vi "HDF5_Test9-openFile.vi"() -> ()   [LabVIEW 2018]
uses:
  <vilib>/addons/h5labview2/base/h5o_type.ctl
  HDF5/HDF5_NoiseInfoClust.ctl
  <vilib>/addons/h5labview2/file/H5Fmode.ctl
  HDF5/lib_path_mod_20200519.vi
  <vilib>/addons/h5labview2/base/H5Equery.vi
  <vilib>/addons/h5labview2/dataset/H5Dread.llb/H5Dread.xnode
  <vilib>/addons/h5labview2/file/H5F.lvlib
  <vilib>/addons/h5labview2/group/H5G.lvlib
  <vilib>/addons/h5labview2/base/hid_t_renamed.ctl
panel:
  out "data 2":T1[][](array[typedef]) {"Sum" format="%^#.1g"}
  out "types 2":T2[](array[typedef])
  out "element":string
  out "data":T1={"Timestring"="", "Timestamp"=0.0, "df"=7629.39453125, "Sum"=0.0} {"Sum" format="%^#.1g"}
  out "found?":bool
  out "names 2":string[](array[string])
  in  "index":i32
  in  "path":path
  out "types":T2[](array[typedef])
  out "names":string[](array[string])
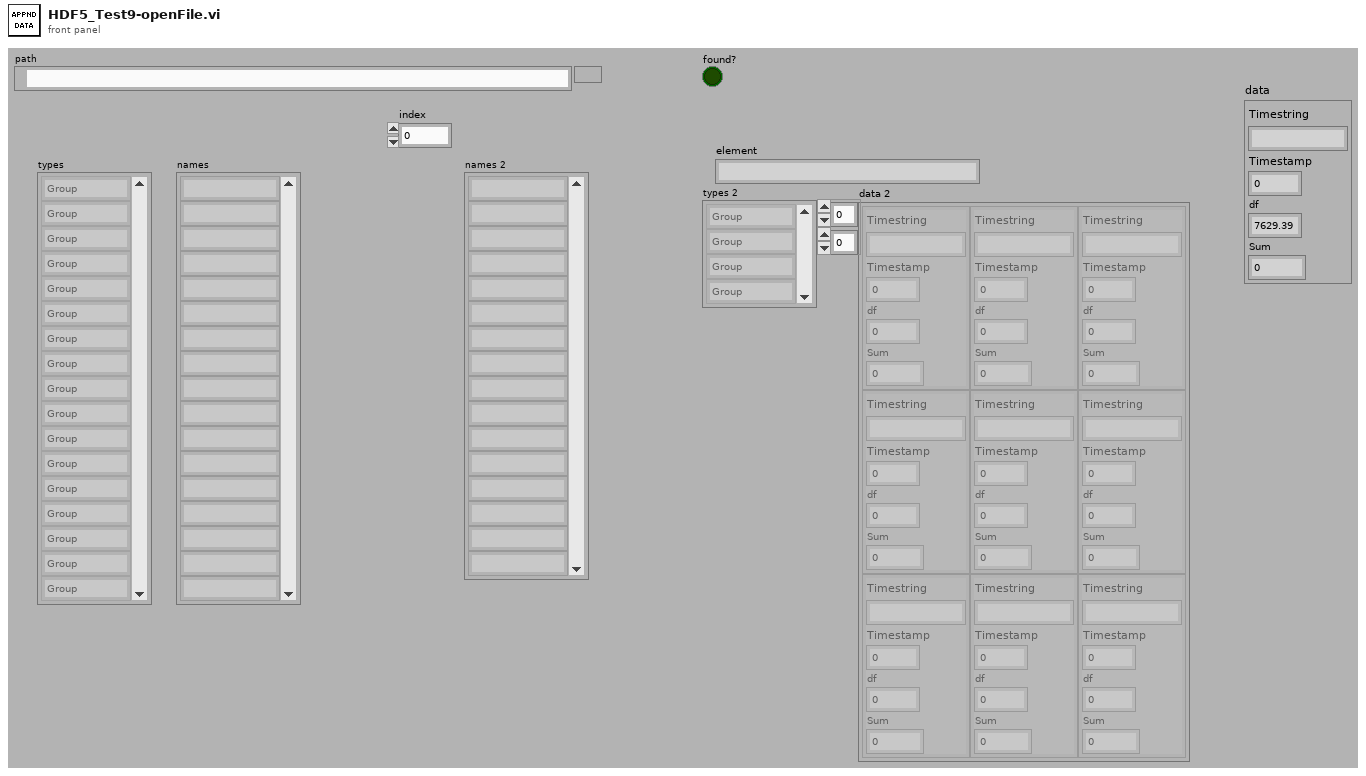
[diagram p1: front panel]
types:
  T1 = typedef "HDF5_NoiseInfoClust.ctl" = cluster{"Timestring":string, "Timestamp":dbl, "df":dbl, "Sum":dbl}
  T2 = typedef "h5o_type.ctl" = enum8{"Group", "Dataset", "Named type"}
  T3 = typedef "H5F.lvlib/H5Fmode.ctl" = enum16{"read-only", "read-write", "overwrite", "create new", "open or create"}
  T4 = typedef "hid_t.ctl" = i32
  T5 = typedef "HDF5_ToneInfoClust.ctl" = cluster{"Timestring":string, "Timestamp":dbl, "MaxValue":dbl, "PeakLoc":dbl, "df":dbl}
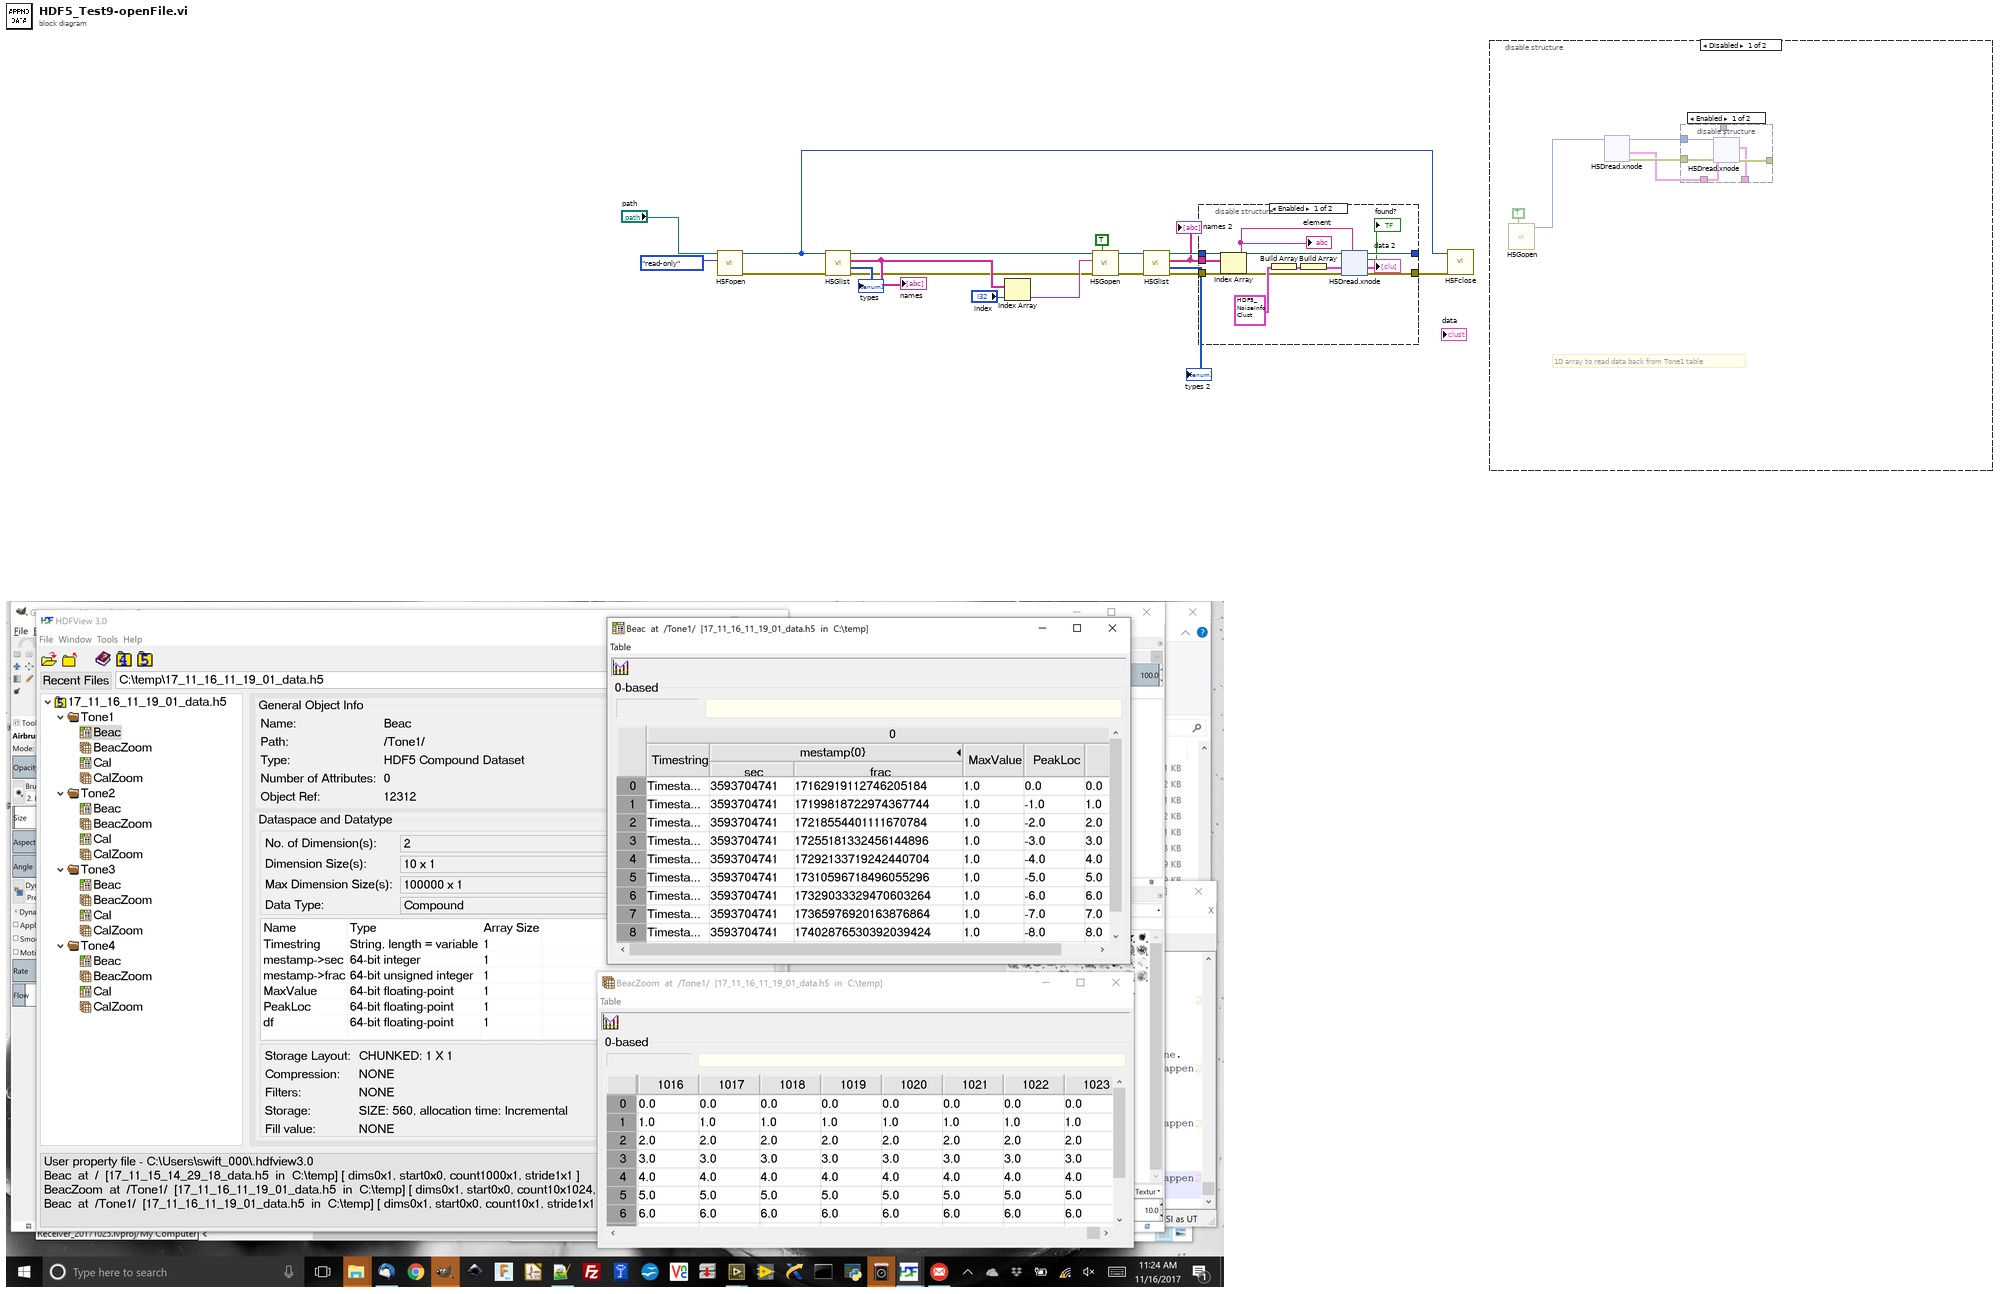
[diagram p0: block diagram]
diagram:
  n1 = call <vilib>:"H5Fopen.vi"("mode (read-only)"=H5Fmode."read-only" ("mode"), "path"="path") -> ("error out"=w15:errorcluster, "ref out"=w7:T4)  [unwired: 8 in]
  n2 = call <vilib>:"H5Glist.vi"("error in (no error)"=w15, "ref in"=w7) -> ("error out"=w6:errorcluster, "types"=→"types":T2[], "names"=w12:string[], "ref out"=w13:T4)  [unwired: 6 in]
  "names" <- w12
  n3 = Index Array(array=w12, index="index") -> (element=w10:string)
  n4 = call <vilib>:"H5Gopen.vi"("create? (F)"=TRUE, "error in (no error)"=w6, "name"=w10, "ref in"=w13) -> ("error out"=w5:errorcluster, "group out"=w9:T4)  [unwired: 6 in]
  n5 = call <vilib>:"H5Glist.vi"("error in (no error)"=w5, "ref in"=w9) -> ("error out"=w3:errorcluster, "types"=→"types 2":T2[], "names"=w4:string[], "ref out"=w8:T4)  [unwired: 6 in]
  "names 2" <- w4
  n6 = disable-structure shown="Enabled" {
    disable-tunnel: w4 -> [w29 _]
    disable-tunnel: w8 -> [w28 _]
    disable-tunnel: [w26 _] -> _
    disable-tunnel: w3 -> [w23 w45]
    disable-tunnel: [w22 w45] -> w2
    frame Enabled {
      n7 = Index Array(array=w29) -> (element=w27:string)  [unwired: 1 in]
      "element" <- w27
      n8 = Build Array(T1 {"Timestring"="Timestamp string goes here", "Timestamp"=0.0, "df"=7629.39453125, "Sum"=0.0} ("HDF5_NoiseInfo")) -> (w21:T1[])
      n9 = Build Array(w21) -> (w20:T1[][])
      n10 = xnode "H5Dread.xnode"("dataset name (this)"=w27, "error in (no error)"=w23, "default"=w20, "ref in"=w28) -> ("error out"=w22:errorcluster, "data"=→"data 2":T1[][], "found?"=→"found?":bool, "ref out"=w26:i32)  [unwired: 2 in]
    }
    frame Disabled {
    }
  }
  n11 = call <vilib>:"H5Fclose.vi"("error in (no error)"=w2, "ref"=w7) -> ()  [unwired: 9 in, 1 out]
  n12 = disable-structure shown="Disabled" {
    frame Disabled {
      # "1D array to read data back from Tone1 table"
      n13 = call <vilib>:"H5Gopen.vi"("create? (F)"=TRUE) -> ("group out"=w46:T4)  [unwired: 9 in, 1 out]
      n14 = xnode "H5Dread.xnode"("ref in"=w46) -> ("error out"=w49:errorcluster, "ref out"=w50:i32, "default"=w48:T5[])  [unwired: 4 in, 2 out]
      n15 = disable-structure shown="Enabled" {
        disable-tunnel: w50 -> [w56 _]
        disable-tunnel: _ -> [w55 _]
        disable-tunnel: w49 -> [w54 w72]
        disable-tunnel: [w53 w72] -> _
        disable-tunnel: w48 -> [w52 _]
        disable-tunnel: [w51 _] -> _
        frame Enabled {
          n16 = xnode "H5Dread.xnode"("dataset name (this)"=w55, "error in (no error)"=w54, "default"=w52, "ref in"=w56) -> ("error out"=w53:errorcluster, "data"=w51:T5[])  [unwired: 2 in, 2 out]
        }
        frame Disabled {
        }
      }
    }
    frame Enabled {
    }
  }
